vi "DofType2IndexesAndSpace.vi"(11 "DofType":T3=enum."Cartesian Forces & Moments") -> (1 "Fault Type":T1, 3 "Space Type":T2)   [LabVIEW 2009]
uses:
  Data Access Objects/Limits/DofTypes.ctl
  Space Type.ctl
  Fault Type.ctl
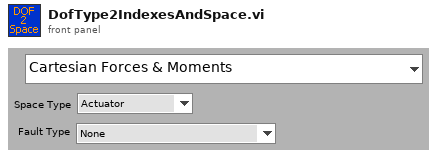
[diagram p1: front panel]
types:
  T1 = typedef "Fault Type.ctl" = enum16{"None", "Command", "Displacement", "Force", "Increment"}
  T2 = typedef "Space Type.ctl" = enum16{"Actuator", "Cartesian"}
  T3 = typedef "DofTypes.ctl" = enum16{"Cartesian Displacements", "Cartesian Forces & Moments", "Actuator Displacements", "Actuator Forces", "Cartesian Increments", "Actuator Increments"}
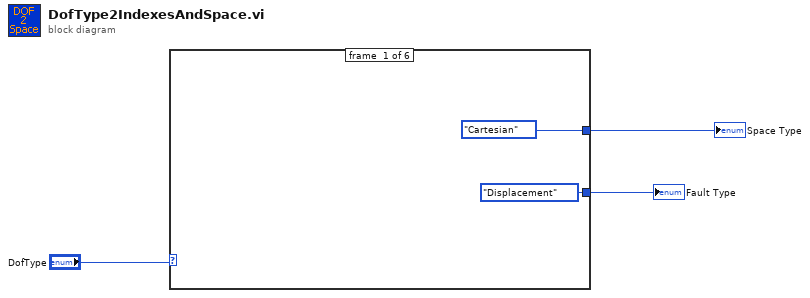
[diagram p0: block diagram]
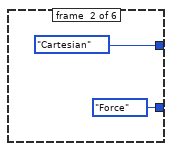
[diagram p2: hidden frame]
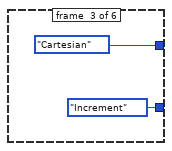
[diagram p3: hidden frame]
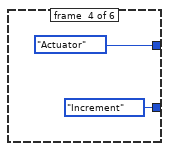
[diagram p4: hidden frame]
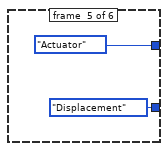
[diagram p5: hidden frame]
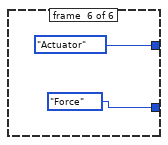
[diagram p6: hidden frame]
diagram:
  n1 = case shown="\"Actuator Increments\"" "DofType" {
    tunnel: [Space_Type."Cartesian" ("Space Type") Space_Type."Cartesian" ("Space Type") Space_Type."Cartesian" ("Space Type") Space_Type."Actuator" ("Space Type") Space_Type."Actuator" ("Space Type") Space_Type."Actuator" ("Space Type")] -> w2
    tunnel: [Fault_Type."Displacement" ("Fault Type") Fault_Type."Force" ("Fault Type") Fault_Type."Increment" ("Fault Type") Fault_Type."Increment" ("Fault Type") Fault_Type."Displacement" ("Fault Type") Fault_Type."Force" ("Fault Type")] -> w1
    frame #0 {
    }
    frame #1 {
    }
    frame #2 {
    }
    frame #3 {
    }
    frame #4 {
    }
    frame #5 {
    }
  }
  "Space Type" <- w2
  "Fault Type" <- w1
